vi "PROJETO OK.vi"() -> ()   [LabVIEW 2018]
uses:
  <vilib>/Instr/_visa.llb/VISA Configure Serial Port (Instr).vi
panel:
  out "LED High":bool
  out "LED Med":bool
  out "LED Low":bool
  out "Status Arduíno":string
  out "read buffer":string
  out "X1":i32
  out "Y1":i32
  out "X2":i32
  out "Y2":i32
  out "Torre 1":T1(graph)
  out "Torre 2":T1(graph)
  in  "Enviar":bool
  in  "Rápido":bool
  in  "Normal":bool
  in  "Devagar":bool
  out "Dados enviados":string
  out "Status motor":string
  in  "stop":bool
  in  "Porta de comunicação":refnum<visa-resource-name>
  in  "Power":bool
  # "Sistema de Monitoramento do Amortecimento \nde uma estrutura através de contrapeso inercial"
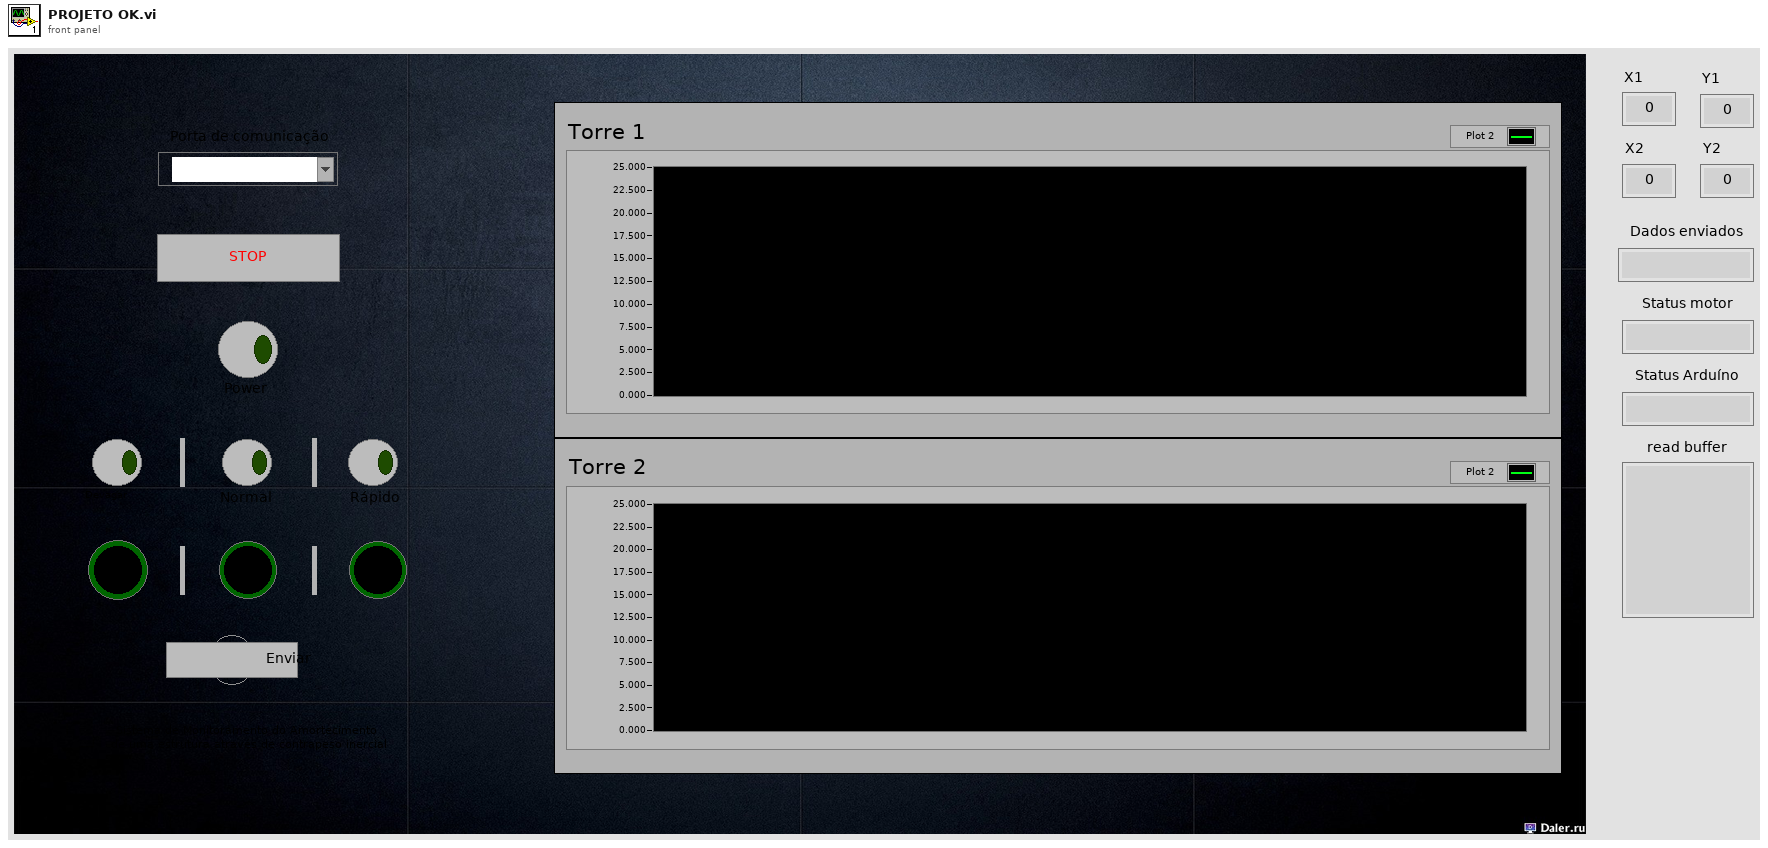
[diagram p1: front panel]
types:
  T1 = cluster{"offset past number":i32, "offset past number":i32}
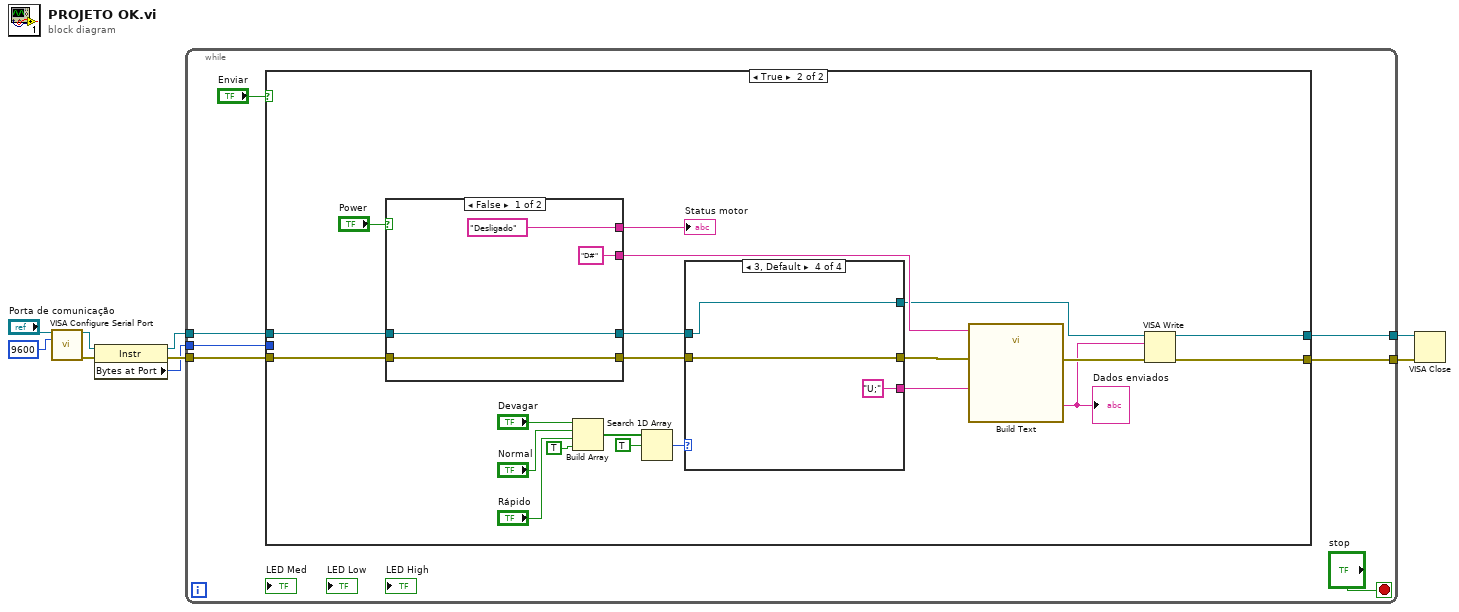
[diagram p0: block diagram]
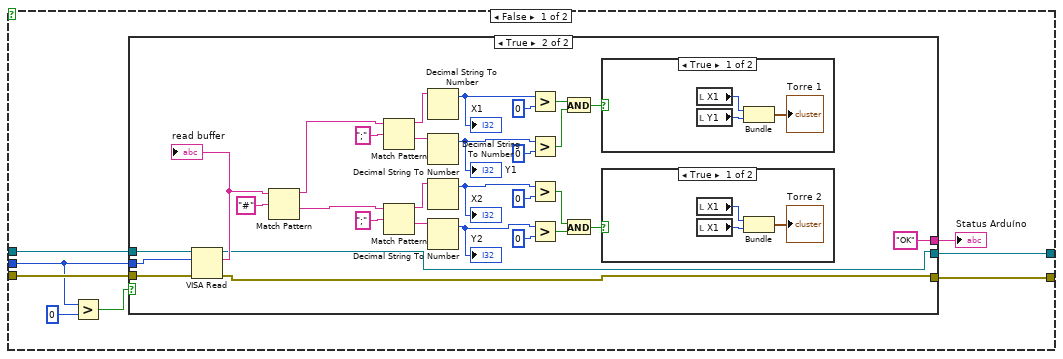
[diagram p2: hidden frame]
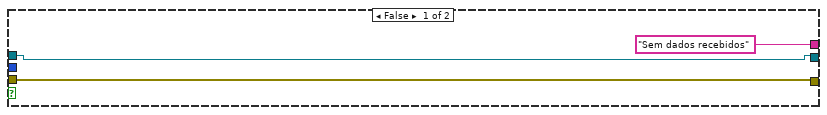
[diagram p3: hidden frame]
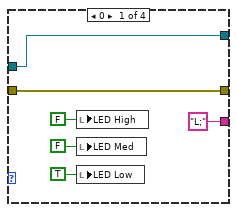
[diagram p6: hidden frame]
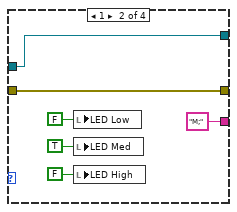
[diagram p7: hidden frame]
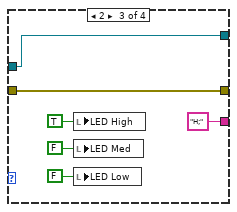
[diagram p8: hidden frame]
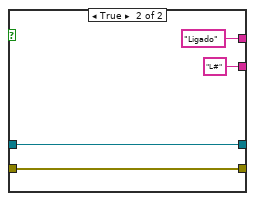
[diagram p9: hidden frame]
diagram:
  n1 = call-poly "VISA Configure Serial Port"("VISA resource name"="Porta de comunicação", "baud rate (9600)"=u32 9600) -> ("VISA resource name out"=w8:refnum<visa-resource-name>, "error out"=w7:errorcluster)  [unwired: 12 in]
  n2 = property class="Instr"(reference=w8, error in=w7) -> (reference out=w5:refnum<visa-resource-name>, error out=w6:errorcluster, "Bytes at Port"=w4:u32)
  n3 = while {
    tunnel: w5 -> [w14]
    tunnel: w6 -> [w15]
    tunnel: w4 -> [w12]
    tunnel: [w11] -> w3
    tunnel: [w10] -> w2
    stop <- "stop" stop-if-true
    n4 = case shown="True" "Enviar" {
      tunnel: w15 -> [w22 w66]
      tunnel: w14 -> [w23 w67]
      tunnel: w12 -> [w19 _]
      tunnel: [w21 w65] -> w11
      tunnel: [w17 w64] -> w10
      frame False {
        n5 = Greater?(x=w19, y=u32 0) -> (0:w18:bool)
        n6 = case shown="True" w18 {
          tunnel: ["Sem dados recebidos" ("Status Arduíno") "OK" ("Status Arduíno")] -> w24
          tunnel: [w25 w46] -> w17
          tunnel: [w26 w31] -> w21
          tunnel: w23 -> [w26 w30]
          tunnel: w22 -> [w25 w29]
          tunnel: w19 -> [_ w28]
          frame False {
          }
          frame True {
            n7 = VISA Read(VISA resource name=w30, byte count=w28, error in (no error)=w29) -> (VISA resource name out=w31:refnum<visa-resource-name>, read buffer=w57:string, error out=w46:errorcluster)  [unwired: 1 out]
            "read buffer" <- w57
            n8 = Match Pattern(string=w57, regular expression="#") -> (before substring=w55:string, after substring=w52:string)  [unwired: 1 in, 2 out]
            n9 = Match Pattern(string=w55, regular expression=";") -> (before substring=w51:string, after substring=w50:string)  [unwired: 1 in, 2 out]
            n10 = Match Pattern(string=w52, regular expression=";") -> (before substring=w49:string, after substring=w48:string)  [unwired: 1 in, 2 out]
            n11 = Decimal String To Number(string=w51) -> (offset past number=w45:i32)  [unwired: 2 in, 1 out]
            "X1" <- w45
            n12 = Decimal String To Number(string=w50) -> (offset past number=w40:i32)  [unwired: 2 in, 1 out]
            "Y1" <- w40
            n13 = Decimal String To Number(string=w49) -> (offset past number=w39:i32)  [unwired: 2 in, 1 out]
            "X2" <- w39
            n14 = Decimal String To Number(string=w48) -> (offset past number=w38:i32)  [unwired: 2 in, 1 out]
            "Y2" <- w38
            n15 = Greater?(x=w45, y=u32 0) -> (0:w37:bool)
            n16 = Greater?(x=w40, y=u32 0) -> (0:w36:bool)
            n17 = Greater?(x=w39, y=u32 0) -> (0:w35:bool)
            n18 = Greater?(x=w38, y=u32 0) -> (0:w34:bool)
            n19 = And(x=w37, y=w36) -> (x .and. y?=w33:bool)
            n20 = And(x=w35, y=w34) -> (x .and. y?=w32:bool)
            n21 = case shown="True" w33 {
              frame True {
                n22 = local read "X1"() -> (w63:i32)
                n23 = local read "Y1"() -> (w62:i32)
                n24 = Bundle("X1"=w63, "Y1"=w62) -> (→"Torre 1":cluster{"X1":i32, "Y1":i32})  [unwired: 1 in]
              }
              frame False {
              }
            }
            n25 = case shown="True" w32 {
              frame True {
                n26 = local read "X1"() -> (w60:i32)
                n27 = local read "X1"() -> (w59:i32)
                n28 = Bundle("X1"=w60, "X1"=w59) -> (→"Torre 2":cluster{"X1":i32, "X1":i32})  [unwired: 1 in]
              }
              frame False {
              }
            }
          }
        }
        "Status Arduíno" <- w24
      }
      frame True {
        n29 = case shown="False" "Power" {
          tunnel: w67 -> [w109 w112]
          tunnel: w66 -> [w108 w111]
          tunnel: [w109 w112] -> w81
          tunnel: [w108 w111] -> w82
          tunnel: ["Desligado" "Ligado"] -> w80
          tunnel: ["D#" ("write buffer") "L#" ("write buffer")] -> w79
          frame False {
          }
          frame True {
          }
        }
        "Status motor" <- w80
        n30 = Build Array("Devagar", "Normal", "Rápido", TRUE ("element")) -> (w84:bool[])
        n31 = Search 1D Array(1D array=w84, element=TRUE) -> (index of element=w83:i32)  [unwired: 1 in]
        n32 = case shown="3, Default" w83 {
          tunnel: w82 -> [w89 w95 w100 w105]
          tunnel: w81 -> [w90 w96 w102 w104]
          tunnel: [w90 w96 w102 w104] -> w69
          tunnel: [w89 w95 w100 w105] -> w72
          tunnel: ["L;" ("write buffer") "M;" ("write buffer") "H;" ("write buffer") "U;" ("write buffer")] -> w78
          frame 0 {
            n33 = local write "LED High"(FALSE ("Med")) -> ()
            n34 = local write "LED Med"(FALSE ("High")) -> ()
            n35 = local write "LED Low"(TRUE ("Low")) -> ()
          }
          frame 1 {
            n36 = local write "LED Low"(FALSE ("Low")) -> ()
            n37 = local write "LED Med"(TRUE ("Med")) -> ()
            n38 = local write "LED High"(FALSE ("High")) -> ()
          }
          frame 2 {
            n39 = local write "LED High"(TRUE ("High")) -> ()
            n40 = local write "LED Med"(FALSE ("Med")) -> ()
            n41 = local write "LED Low"(FALSE ("Low")) -> ()
          }
          frame 3, Default {
          }
        }
        n42 = call "Build Text"("Beginning Text"=w79, "parameter1"=w78, "error in (no error)"=w72) -> ("Result"=w70:string, "error out"=w71:errorcluster)  [unwired: 11 in]
        "Dados enviados" <- w70
        n43 = VISA Write(VISA resource name=w69, write buffer=w70, error in (no error)=w71) -> (VISA resource name out=w65:refnum<visa-resource-name>, error out=w64:errorcluster)  [unwired: 1 out]
      }
    }
  }
  n44 = VISA Close(VISA resource name=w3, error in (no error)=w2) -> ()  [unwired: 1 out]
